vi "hit judge.vi"(6 "keys pressed":T1(array[ring]), 7 "click last frame":T1(array[ring]), 8 "hold note key":T2, 9 "score info":T3, 10 "next note":cluster{"1st rail":i32, "2nd rail":i32}, 11 "song info":T4) -> (0 "hold note key":T2, 1 "new score info":T3, 2 "next note":cluster{"1st rail":i32, "2nd rail":i32}, 3 "note acc":cluster{i32, i32})   [LabVIEW 2023]
panel:
  out "keys pressed 2":T1(array[ring])
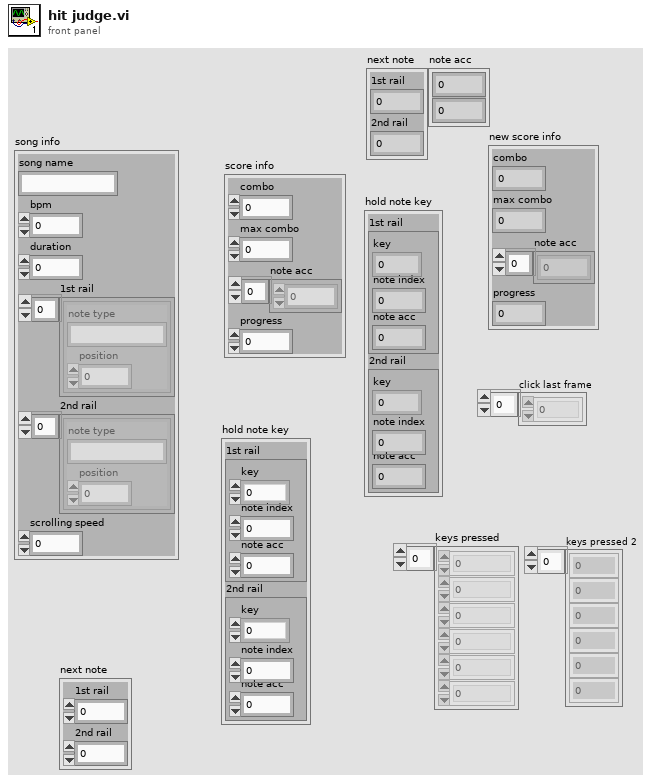
[diagram p1: front panel]
types:
  T1 = enum16{"0", "1", "2", "3", "4", "5", "6", "7", "8", "9", "A", "B", "C", "D", "E", "F", "G", "H", "I", "J", "K", "L", "M", "N", "O", "P", "Q", "R", "S", "T", "U", "V", "W", "X", "Y", "Z", "F1", "F2", "F3", "F4", "F5", "F6", "F7", "F8", "F9", "F10", "F11", "F12", "F13", "F14", "F15", "ADD", "BACK", "BACKSLASH", "CAPITAL", "COMMA", "DECIMAL", "DELETE", "DIVIDE", "DOWN", "END", "EQUALS", "ESCAPE", "GRAVE (`)", "HOME", "INSERT", "LBRACKET", "LCONTROL", "LEFT", "L ALT", "LSHIFT", "LWIN", "MINUS", "MULTIPLY", "NEXT", "NUMLOCK", "NUMPAD_0", "NUMPAD_1", "NUMPAD_2", "NUMPAD_3", "NUMPAD_4", "NUMPAD_5", "NUMPAD_6", "NUMPAD_7", "NUMPAD_8", "NUMPAD_9", "PAUSE", "PERIOD", "PRIOR (PG UP)", "RBRACKET", "RCONTROL", "RETURN", "RIGHT", "R ALT", "RSHIFT", "RWIN", "SCROLL", "SEMICOLON", "SLASH", "SPACE", "SUBTRACT", "TAB", "UP", "ENTER (num pad)", "' (quote)"}[]
  T2 = cluster{"1st rail":cluster{"key":enum16{"0", "1", "2", "3", "4", "5", "6", "7", "8", "9", "A", "B", "C", "D", "E", "F", "G", "H", "I", "J", "K", "L", "M", "N", "O", "P", "Q", "R", "S", "T", "U", "V", "W", "X", "Y", "Z", "F1", "F2", "F3", "F4", "F5", "F6", "F7", "F8", "F9", "F10", "F11", "F12", "F13", "F14", "F15", "ADD", "BACK", "BACKSLASH", "CAPITAL", "COMMA", "DECIMAL", "DELETE", "DIVIDE", "DOWN", "END", "EQUALS", "ESCAPE", "GRAVE (`)", "HOME", "INSERT", "LBRACKET", "LCONTROL", "LEFT", "L ALT", "LSHIFT", "LWIN", "MINUS", "MULTIPLY", "NEXT", "NUMLOCK", "NUMPAD_0", "NUMPAD_1", "NUMPAD_2", "NUMPAD_3", "NUMPAD_4", "NUMPAD_5", "NUMPAD_6", "NUMPAD_7", "NUMPAD_8", "NUMPAD_9", "PAUSE", "PERIOD", "PRIOR (PG UP)", "RBRACKET", "RCONTROL", "RETURN", "RIGHT", "R ALT", "RSHIFT", "RWIN", "SCROLL", "SEMICOLON", "SLASH", "SPACE", "SUBTRACT", "TAB", "UP", "ENTER (num pad)", "' (quote)"}, "note index":i32, "note acc":i32}, "2nd rail":cluster{"key":enum16{"0", "1", "2", "3", "4", "5", "6", "7", "8", "9", "A", "B", "C", "D", "E", "F", "G", "H", "I", "J", "K", "L", "M", "N", "O", "P", "Q", "R", "S", "T", "U", "V", "W", "X", "Y", "Z", "F1", "F2", "F3", "F4", "F5", "F6", "F7", "F8", "F9", "F10", "F11", "F12", "F13", "F14", "F15", "ADD", "BACK", "BACKSLASH", "CAPITAL", "COMMA", "DECIMAL", "DELETE", "DIVIDE", "DOWN", "END", "EQUALS", "ESCAPE", "GRAVE (`)", "HOME", "INSERT", "LBRACKET", "LCONTROL", "LEFT", "L ALT", "LSHIFT", "LWIN", "MINUS", "MULTIPLY", "NEXT", "NUMLOCK", "NUMPAD_0", "NUMPAD_1", "NUMPAD_2", "NUMPAD_3", "NUMPAD_4", "NUMPAD_5", "NUMPAD_6", "NUMPAD_7", "NUMPAD_8", "NUMPAD_9", "PAUSE", "PERIOD", "PRIOR (PG UP)", "RBRACKET", "RCONTROL", "RETURN", "RIGHT", "R ALT", "RSHIFT", "RWIN", "SCROLL", "SEMICOLON", "SLASH", "SPACE", "SUBTRACT", "TAB", "UP", "ENTER (num pad)", "' (quote)"}, "note index":i32, "note acc":i32}}
  T3 = cluster{"combo":i32, "max combo":i32, "note acc":i32[], "progress":dbl}
  T4 = cluster{"song name":string, "bpm":i32, "duration":i32, "1st rail":cluster{"note type":string, "position":dbl}[], "2nd rail":cluster{"note type":string, "position":dbl}[], "scrolling speed":dbl}
  T5 = enum16{"0", "1", "2", "3", "4", "5", "6", "7", "8", "9", "A", "B", "C", "D", "E", "F", "G", "H", "I", "J", "K", "L", "M", "N", "O", "P", "Q", "R", "S", "T", "U", "V", "W", "X", "Y", "Z", "F1", "F2", "F3", "F4", "F5", "F6", "F7", "F8", "F9", "F10", "F11", "F12", "F13", "F14", "F15", "ADD", "BACK", "BACKSLASH", "CAPITAL", "COMMA", "DECIMAL", "DELETE", "DIVIDE", "DOWN", "END", "EQUALS", "ESCAPE", "GRAVE (`)", "HOME", "INSERT", "LBRACKET", "LCONTROL", "LEFT", "L ALT", "LSHIFT", "LWIN", "MINUS", "MULTIPLY", "NEXT", "NUMLOCK", "NUMPAD_0", "NUMPAD_1", "NUMPAD_2", "NUMPAD_3", "NUMPAD_4", "NUMPAD_5", "NUMPAD_6", "NUMPAD_7", "NUMPAD_8", "NUMPAD_9", "PAUSE", "PERIOD", "PRIOR (PG UP)", "RBRACKET", "RCONTROL", "RETURN", "RIGHT", "R ALT", "RSHIFT", "RWIN", "SCROLL", "SEMICOLON", "SLASH", "SPACE", "SUBTRACT", "TAB", "UP", "ENTER (num pad)", "' (quote)"}
  T6 = cluster{"key":enum16{"0", "1", "2", "3", "4", "5", "6", "7", "8", "9", "A", "B", "C", "D", "E", "F", "G", "H", "I", "J", "K", "L", "M", "N", "O", "P", "Q", "R", "S", "T", "U", "V", "W", "X", "Y", "Z", "F1", "F2", "F3", "F4", "F5", "F6", "F7", "F8", "F9", "F10", "F11", "F12", "F13", "F14", "F15", "ADD", "BACK", "BACKSLASH", "CAPITAL", "COMMA", "DECIMAL", "DELETE", "DIVIDE", "DOWN", "END", "EQUALS", "ESCAPE", "GRAVE (`)", "HOME", "INSERT", "LBRACKET", "LCONTROL", "LEFT", "L ALT", "LSHIFT", "LWIN", "MINUS", "MULTIPLY", "NEXT", "NUMLOCK", "NUMPAD_0", "NUMPAD_1", "NUMPAD_2", "NUMPAD_3", "NUMPAD_4", "NUMPAD_5", "NUMPAD_6", "NUMPAD_7", "NUMPAD_8", "NUMPAD_9", "PAUSE", "PERIOD", "PRIOR (PG UP)", "RBRACKET", "RCONTROL", "RETURN", "RIGHT", "R ALT", "RSHIFT", "RWIN", "SCROLL", "SEMICOLON", "SLASH", "SPACE", "SUBTRACT", "TAB", "UP", "ENTER (num pad)", "' (quote)"}, "note index":i32, "note acc":i32}
  T7 = cluster{"element":enum16{"0", "1", "2", "3", "4", "5", "6", "7", "8", "9", "A", "B", "C", "D", "E", "F", "G", "H", "I", "J", "K", "L", "M", "N", "O", "P", "Q", "R", "S", "T", "U", "V", "W", "X", "Y", "Z", "F1", "F2", "F3", "F4", "F5", "F6", "F7", "F8", "F9", "F10", "F11", "F12", "F13", "F14", "F15", "ADD", "BACK", "BACKSLASH", "CAPITAL", "COMMA", "DECIMAL", "DELETE", "DIVIDE", "DOWN", "END", "EQUALS", "ESCAPE", "GRAVE (`)", "HOME", "INSERT", "LBRACKET", "LCONTROL", "LEFT", "L ALT", "LSHIFT", "LWIN", "MINUS", "MULTIPLY", "NEXT", "NUMLOCK", "NUMPAD_0", "NUMPAD_1", "NUMPAD_2", "NUMPAD_3", "NUMPAD_4", "NUMPAD_5", "NUMPAD_6", "NUMPAD_7", "NUMPAD_8", "NUMPAD_9", "PAUSE", "PERIOD", "PRIOR (PG UP)", "RBRACKET", "RCONTROL", "RETURN", "RIGHT", "R ALT", "RSHIFT", "RWIN", "SCROLL", "SEMICOLON", "SLASH", "SPACE", "SUBTRACT", "TAB", "UP", "ENTER (num pad)", "' (quote)"}, i32, i32}
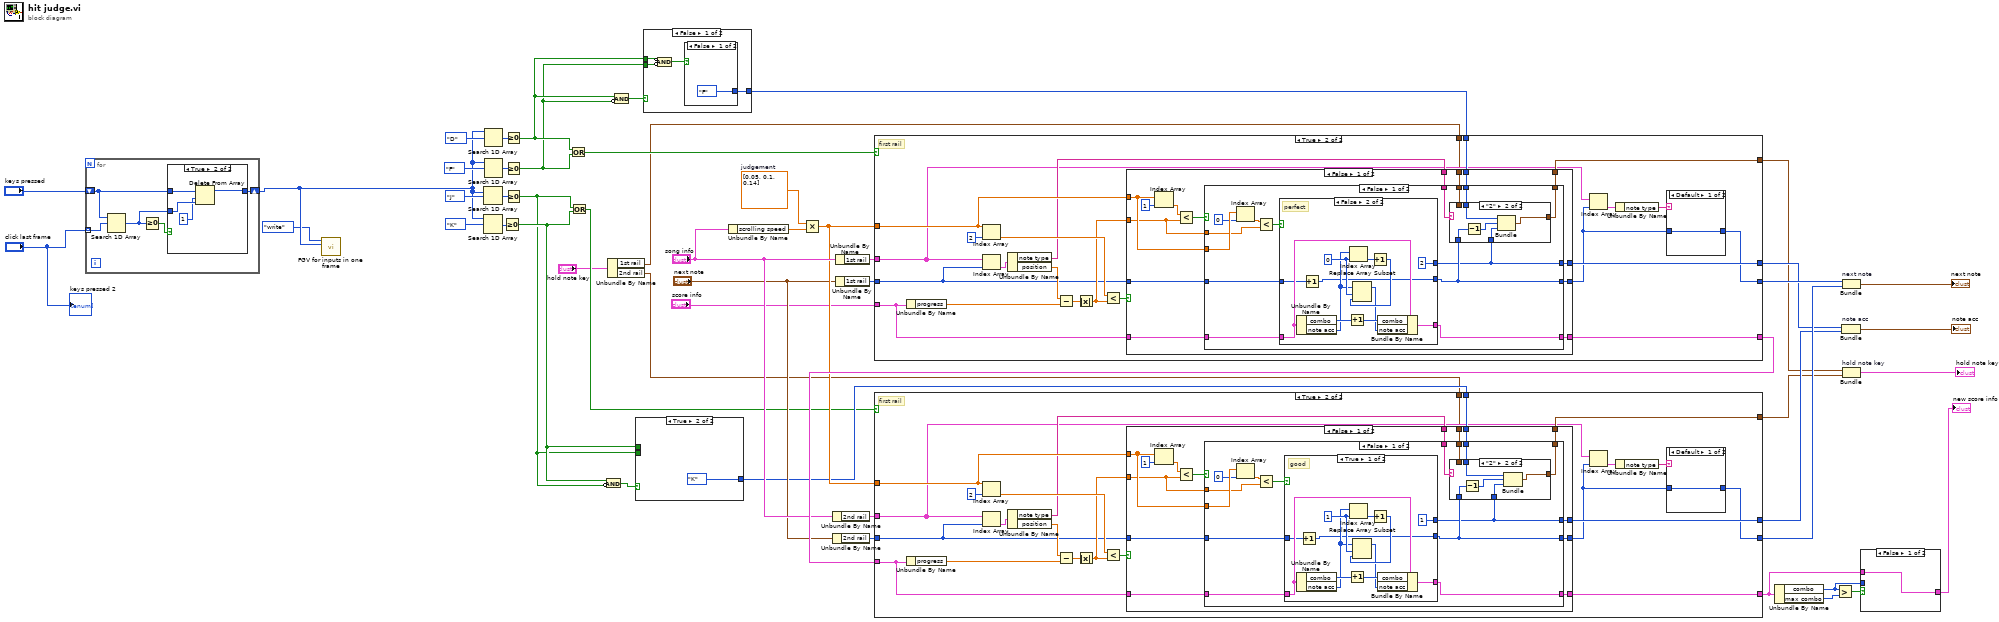
[diagram p0: block diagram]
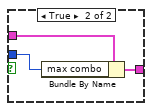
[diagram p3: hidden frame]
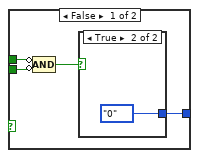
[diagram p4: hidden frame]
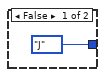
[diagram p5: hidden frame]
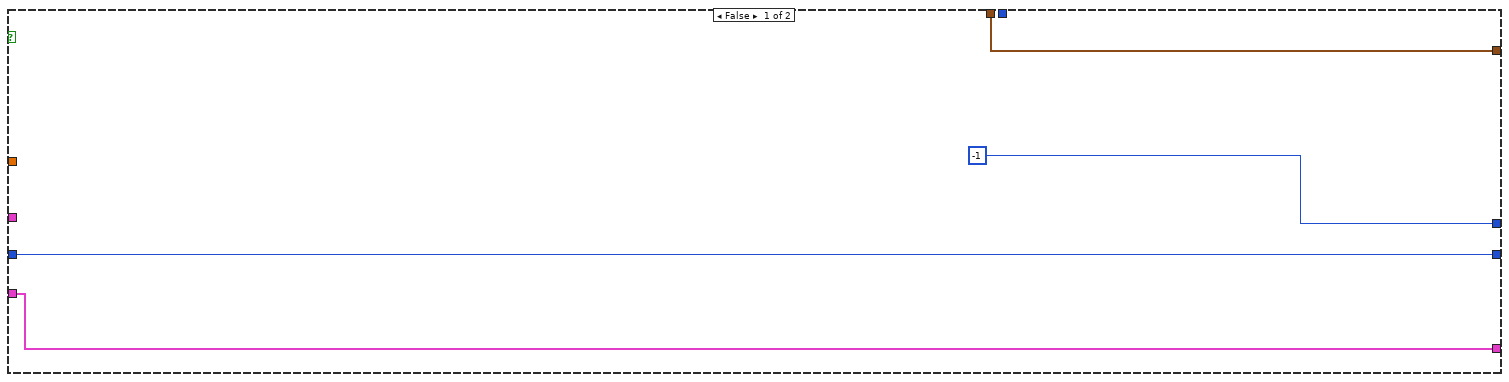
[diagram p6: hidden frame]
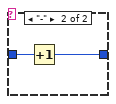
[diagram p7: hidden frame]
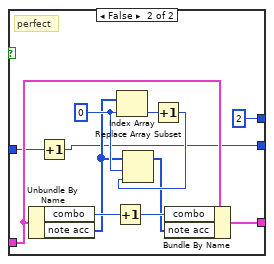
[diagram p9: hidden frame]
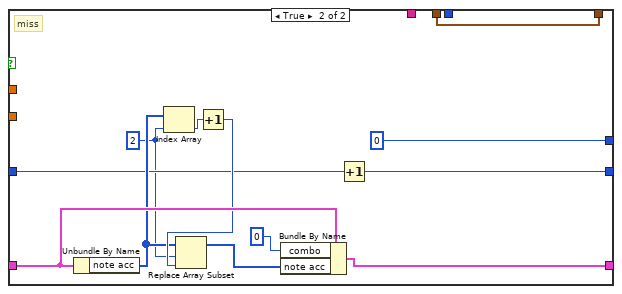
[diagram p10: hidden frame]
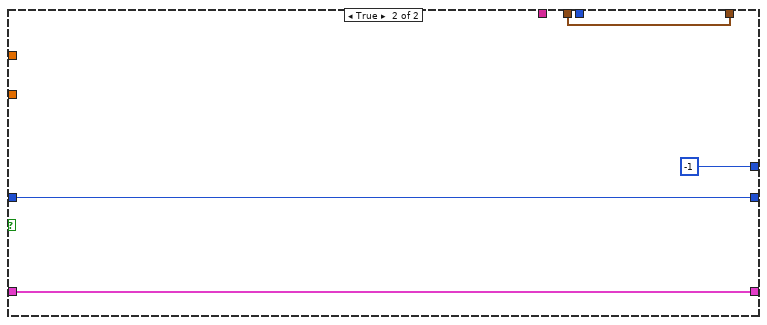
[diagram p11: hidden frame]
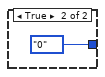
[diagram p12: hidden frame]
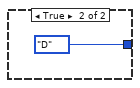
[diagram p13: hidden frame]
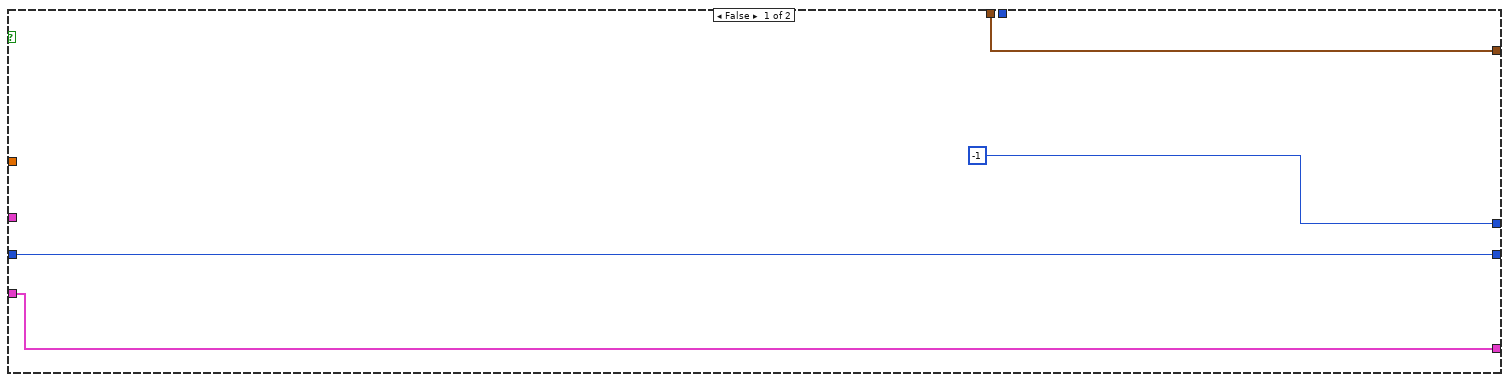
[diagram p14: hidden frame]
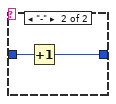
[diagram p15: hidden frame]
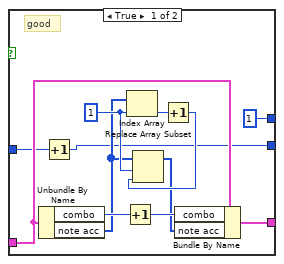
[diagram p17: hidden frame]
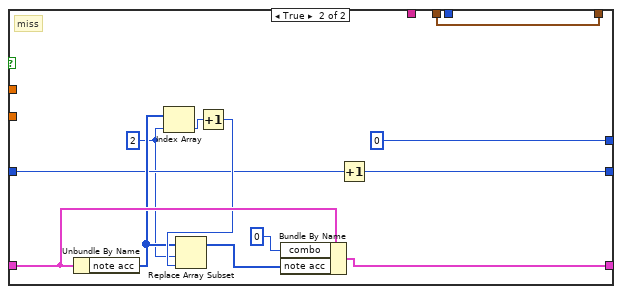
[diagram p18: hidden frame]
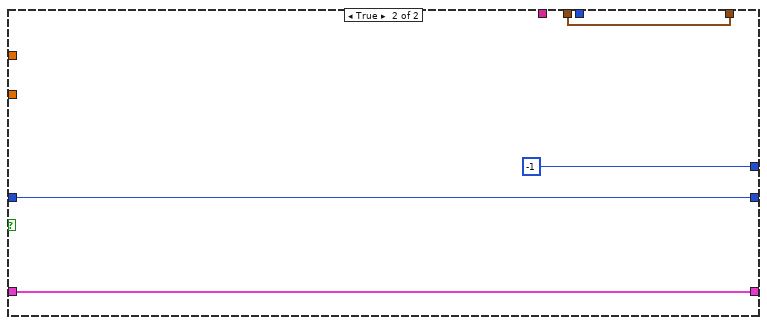
[diagram p19: hidden frame]
diagram:
  w49 = dbl[] [0.05, 0.1, 0.14]  # judgement
  n1 = for {
    tunnel: "click last frame" -> [w55] mode=indexing
    shift-right: [w52] -> w3
    shift-left: "keys pressed" -> [w53]
    n2 = Search 1D Array(1D array=w53, element=w55) -> (index of element=w51:i32)  [unwired: 1 in]
    n3 = Greater Or Equal To 0?(x=w51) -> (x >= 0?=w54:bool)
    n4 = case shown="True" w54 {
      tunnel: w53 -> [w56 w60]
      tunnel: [w56 w59] -> w52
      tunnel: w51 -> [_ w58]
      frame False {
      }
      frame True {
        n5 = Delete From Array(array=w60, length=1, index=w58) -> (array with subset deleted=w59:T1)  [unwired: 1 out]
      }
    }
  }
  n6 = call "FGV for inputs in one frame.vi"("write in key"=w3, "mode"=enum16{"read", "write"}."write") -> ()  [unwired: 9 in, 1 out]
  n7 = Search 1D Array(1D array=w3, element=T5."J") -> (index of element=w42:i32)  [unwired: 1 in]
  n8 = Search 1D Array(1D array=w3, element=T5."K") -> (index of element=w41:i32)  [unwired: 1 in]
  n9 = Search 1D Array(1D array=w3, element=T5."D") -> (index of element=w46:i32)  [unwired: 1 in]
  n10 = Search 1D Array(1D array=w3, element=T5."F") -> (index of element=w45:i32)  [unwired: 1 in]
  n11 = Greater Or Equal To 0?(x=w41) -> (x >= 0?=w26:bool)
  n12 = Greater Or Equal To 0?(x=w46) -> (x >= 0?=w37:bool)
  n13 = Greater Or Equal To 0?(x=w45) -> (x >= 0?=w36:bool)
  n14 = Greater Or Equal To 0?(x=w42) -> (x >= 0?=w25:bool)
  n15 = Or(x=w37, y=w36) -> (x .or. y?=w40:bool)
  n16 = Or(x=w25, y=w26) -> (x .or. y?=w23:bool)
  n17 = Compound Arithmetic op=AND(w26, invert w25) -> (w27:bool)
  n18 = Unbundle By Name("hold note key") -> ("1st rail"=w6:T6, "2nd rail"=w5:T6)
  n19 = Compound Arithmetic op=AND(w37, invert w36) -> (w38:bool)
  n20 = case shown="True" w27 {
    tunnel: [w61 T5."K" ("element")] -> w24
    tunnel: w26 -> [w64 _]
    tunnel: w25 -> [w63 _]
    frame False {
      n21 = Compound Arithmetic op=AND(invert w64, invert w63) -> (w62:bool)
      n22 = case shown="True" w62 {
        tunnel: [T5."J" ("element") T5."0" ("element")] -> w61
        frame False {
        }
        frame True {
        }
      }
    }
    frame True {
    }
  }
  n23 = case shown="False" w38 {
    tunnel: [w68 T5."D" ("element")] -> w35
    tunnel: w37 -> [w71 _]
    tunnel: w36 -> [w70 _]
    frame False {
      n24 = Compound Arithmetic op=AND(invert w71, invert w70) -> (w69:bool)
      n25 = case shown="False" w69 {
        tunnel: [T5."F" ("element") T5."0" ("element")] -> w68
        frame False {
        }
        frame True {
        }
      }
    }
    frame True {
    }
  }
  n26 = Unbundle By Name("song info") -> ("scrolling speed"=w50:dbl)
  n27 = Multiply(x=w49, y=w50) -> (x*y=w32:dbl[])
  n28 = Unbundle By Name("song info") -> ("2nd rail"=w28:cluster{"note type":string, "position":dbl}[])
  n29 = Unbundle By Name("next note") -> ("2nd rail"=w30:i32)
  n30 = Unbundle By Name("song info") -> ("1st rail"=w29:cluster{"note type":string, "position":dbl}[])
  n31 = Unbundle By Name("next note") -> ("1st rail"=w39:i32)
  n32 = case shown="True" w40 {
    tunnel: w32 -> [_ w91]
    tunnel: "score info" -> [w78 w93]
    tunnel: [w78 w92] -> w34
    tunnel: [w77 w81] -> w22
    tunnel: w39 -> [w77 w89]
    tunnel: [-1 w88] -> w20
    tunnel: w35 -> [_ w86]
    tunnel: w6 -> [w75 w79]
    tunnel: [w75 w85] -> w18
    tunnel: w29 -> [_ w80]
    frame False {
    }
    frame True {
      # "first rail"
      n33 = Unbundle By Name(w93) -> ("progress"=w97:dbl)
      n34 = Index Array(array=w91, index=2) -> (element=w94:dbl)
      n35 = Index Array(array=w80, index=w89) -> (element=w100:cluster{"note type":string, "position":dbl})
      n36 = Unbundle By Name(w100) -> ("note type"=w87:string, "position"=w98:dbl)
      n37 = Subtract(x=w98, y=w97) -> (x-y=w96:dbl)
      n38 = Absolute Value(x=w96) -> (abs(x)=w90:dbl)
      n39 = Less?(x=w94, y=w90) -> (x < y?=w95:bool)
      n40 = case shown="False" w95 {
        tunnel: w89 -> [w111 w177]
        tunnel: w93 -> [w114 w176]
        tunnel: [w113 w176] -> w92
        tunnel: [w112 w177] -> w82
        tunnel: w91 -> [w110 _]
        tunnel: w90 -> [w109 _]
        tunnel: [w108 -1] -> w88
        tunnel: w87 -> [w107 _]
        tunnel: w86 -> [w106 _]
        tunnel: [w105 w174] -> w85
        tunnel: w79 -> [w104 w174]
        frame False {
          n41 = Index Array(array=w110, index=1) -> (element=w116:dbl)
          n42 = Less?(x=w116, y=w109) -> (x < y?=w115:bool)
          n43 = case shown="False" w115 {
            tunnel: w114 -> [w126 w173]
            tunnel: [w125 w172] -> w113
            tunnel: [w120 w166] -> w112
            tunnel: w111 -> [w124 w165]
            tunnel: w110 -> [w131 _]
            tunnel: w109 -> [w129 _]
            tunnel: [w118 0] -> w108
            tunnel: w107 -> [w123 _]
            tunnel: w106 -> [w122 _]
            tunnel: [w121 w162] -> w105
            tunnel: w104 -> [w119 w162]
            frame False {
              n44 = Index Array(array=w131, index=0) -> (element=w128:dbl)
              n45 = Less?(x=w128, y=w129) -> (x < y?=w127:bool)
              n46 = case shown="False" w127 {
                tunnel: w126 -> [w149 w161]
                tunnel: [w148 w160] -> w125
                tunnel: w124 -> [w140 w152]
                tunnel: [w139 w151] -> w120
                tunnel: [1 2] -> w118
                frame True {
                  w144 = 1
                  # "good"
                  n47 = Unbundle By Name(w149) -> ("combo"=w146:i32, "note acc"=w143:i32[])
                  n48 = Increment(x=w140) -> (x+1=w139:i32)
                  n49 = Increment(x=w146) -> (x+1=w147:i32)
                  n50 = Index Array(array=w143, index=w144) -> (element=w145:i32)
                  n51 = Increment(x=w145) -> (x+1=w142:i32)
                  n52 = Replace Array Subset(array=w143, new element=w142, index=w144) -> (w141:i32[])
                  n53 = Bundle By Name(cluster=w149, "combo"=w147, "note acc"=w141) -> (w148:T3)
                }
                frame False {
                  w156 = 0
                  # "perfect"
                  n54 = Unbundle By Name(w161) -> ("combo"=w158:i32, "note acc"=w155:i32[])
                  n55 = Increment(x=w152) -> (x+1=w151:i32)
                  n56 = Increment(x=w158) -> (x+1=w159:i32)
                  n57 = Index Array(array=w155, index=w156) -> (element=w157:i32)
                  n58 = Increment(x=w157) -> (x+1=w154:i32)
                  n59 = Replace Array Subset(array=w155, new element=w154, index=w156) -> (w153:i32[])
                  n60 = Bundle By Name(cluster=w161, "combo"=w159, "note acc"=w153) -> (w160:T3)
                }
              }
              n61 = case shown="\"2\"" w123 {
                tunnel: [w132 w136] -> w121
                tunnel: w122 -> [_ w134]
                tunnel: w120 -> [_ w137]
                tunnel: w119 -> [w132 _]
                tunnel: w118 -> [_ w133]
                frame Default {
                }
                frame "2" {
                  n62 = Decrement(x=w137) -> (x-1=w135:i32)
                  n63 = Bundle("element"=w134, w135, w133) -> (w136:T7)  [unwired: 1 in]
                }
              }
            }
            frame True {
              w164 = 2 ("new element/subarray")
              # "miss"
              n64 = Unbundle By Name(w173) -> ("note acc"=w168:i32[])
              n65 = Index Array(array=w168, index=w164) -> (element=w170:i32)
              n66 = Increment(x=w170) -> (x+1=w169:i32)
              n67 = Replace Array Subset(array=w168, new element=w169, index=w164) -> (w167:i32[])
              n68 = Bundle By Name(cluster=w173, "combo"=0, "note acc"=w167) -> (w172:T3)
              n69 = Increment(x=w165) -> (x+1=w166:i32)
            }
          }
        }
        frame True {
        }
      }
      n70 = Index Array(array=w80, index=w82) -> (element=w84:cluster{"note type":string, "position":dbl})
      n71 = Unbundle By Name(w84) -> ("note type"=w83:string)
      n72 = case shown="Default" w83 {
        tunnel: w82 -> [w101 w103]
        tunnel: [w101 w102] -> w81
        frame Default {
        }
        frame "-" {
          n73 = Increment(x=w103) -> (x+1=w102:i32)
        }
      }
    }
  }
  n74 = case shown="True" w23 {
    tunnel: w32 -> [_ w194]
    tunnel: w34 -> [w181 w196]
    tunnel: [w181 w195] -> w11
    tunnel: [w180 w184] -> w21
    tunnel: w30 -> [w180 w192]
    tunnel: [-1 w191] -> w19
    tunnel: w24 -> [_ w189]
    tunnel: w5 -> [w178 w182]
    tunnel: [w178 w188] -> w17
    tunnel: w28 -> [_ w183]
    frame False {
    }
    frame True {
      # "first rail"
      n75 = Unbundle By Name(w196) -> ("progress"=w200:dbl)
      n76 = Index Array(array=w194, index=2) -> (element=w197:dbl)
      n77 = Index Array(array=w183, index=w192) -> (element=w203:cluster{"note type":string, "position":dbl})
      n78 = Unbundle By Name(w203) -> ("note type"=w190:string, "position"=w201:dbl)
      n79 = Subtract(x=w201, y=w200) -> (x-y=w199:dbl)
      n80 = Absolute Value(x=w199) -> (abs(x)=w193:dbl)
      n81 = Less?(x=w197, y=w193) -> (x < y?=w198:bool)
      n82 = case shown="False" w198 {
        tunnel: w192 -> [w214 w280]
        tunnel: w196 -> [w217 w279]
        tunnel: [w216 w279] -> w195
        tunnel: [w215 w280] -> w185
        tunnel: w194 -> [w213 _]
        tunnel: w193 -> [w212 _]
        tunnel: [w211 -1] -> w191
        tunnel: w190 -> [w210 _]
        tunnel: w189 -> [w209 _]
        tunnel: [w208 w277] -> w188
        tunnel: w182 -> [w207 w277]
        frame False {
          n83 = Index Array(array=w213, index=1) -> (element=w219:dbl)
          n84 = Less?(x=w219, y=w212) -> (x < y?=w218:bool)
          n85 = case shown="False" w218 {
            tunnel: w217 -> [w229 w276]
            tunnel: [w228 w275] -> w216
            tunnel: [w223 w269] -> w215
            tunnel: w214 -> [w227 w268]
            tunnel: w213 -> [w234 _]
            tunnel: w212 -> [w232 _]
            tunnel: [w221 0] -> w211
            tunnel: w210 -> [w226 _]
            tunnel: w209 -> [w225 _]
            tunnel: [w224 w265] -> w208
            tunnel: w207 -> [w222 w265]
            frame False {
              n86 = Index Array(array=w234, index=0) -> (element=w231:dbl)
              n87 = Less?(x=w231, y=w232) -> (x < y?=w230:bool)
              n88 = case shown="True" w230 {
                tunnel: w229 -> [w252 w264]
                tunnel: [w251 w263] -> w228
                tunnel: w227 -> [w243 w255]
                tunnel: [w242 w254] -> w223
                tunnel: [1 2] -> w221
                frame True {
                  w247 = 1
                  # "good"
                  n89 = Unbundle By Name(w252) -> ("combo"=w249:i32, "note acc"=w246:i32[])
                  n90 = Increment(x=w243) -> (x+1=w242:i32)
                  n91 = Increment(x=w249) -> (x+1=w250:i32)
                  n92 = Index Array(array=w246, index=w247) -> (element=w248:i32)
                  n93 = Increment(x=w248) -> (x+1=w245:i32)
                  n94 = Replace Array Subset(array=w246, new element=w245, index=w247) -> (w244:i32[])
                  n95 = Bundle By Name(cluster=w252, "combo"=w250, "note acc"=w244) -> (w251:T3)
                }
                frame False {
                  w259 = 0
                  # "perfect"
                  n96 = Unbundle By Name(w264) -> ("combo"=w261:i32, "note acc"=w258:i32[])
                  n97 = Increment(x=w255) -> (x+1=w254:i32)
                  n98 = Increment(x=w261) -> (x+1=w262:i32)
                  n99 = Index Array(array=w258, index=w259) -> (element=w260:i32)
                  n100 = Increment(x=w260) -> (x+1=w257:i32)
                  n101 = Replace Array Subset(array=w258, new element=w257, index=w259) -> (w256:i32[])
                  n102 = Bundle By Name(cluster=w264, "combo"=w262, "note acc"=w256) -> (w263:T3)
                }
              }
              n103 = case shown="\"2\"" w226 {
                tunnel: [w235 w237] -> w224
                tunnel: w225 -> [_ w239]
                tunnel: w223 -> [_ w240]
                tunnel: w222 -> [w235 _]
                tunnel: w221 -> [_ w236]
                frame Default {
                }
                frame "2" {
                  n104 = Decrement(x=w240) -> (x-1=w238:i32)
                  n105 = Bundle("element"=w239, w238, w236) -> (w237:T7)  [unwired: 1 in]
                }
              }
            }
            frame True {
              w267 = 2 ("new element/subarray")
              # "miss"
              n106 = Unbundle By Name(w276) -> ("note acc"=w271:i32[])
              n107 = Index Array(array=w271, index=w267) -> (element=w273:i32)
              n108 = Increment(x=w273) -> (x+1=w272:i32)
              n109 = Replace Array Subset(array=w271, new element=w272, index=w267) -> (w270:i32[])
              n110 = Bundle By Name(cluster=w276, "combo"=0, "note acc"=w270) -> (w275:T3)
              n111 = Increment(x=w268) -> (x+1=w269:i32)
            }
          }
        }
        frame True {
        }
      }
      n112 = Index Array(array=w183, index=w185) -> (element=w187:cluster{"note type":string, "position":dbl})
      n113 = Unbundle By Name(w187) -> ("note type"=w186:string)
      n114 = case shown="Default" w186 {
        tunnel: w185 -> [w204 w206]
        tunnel: [w204 w205] -> w184
        frame Default {
        }
        frame "-" {
          n115 = Increment(x=w206) -> (x+1=w205:i32)
        }
      }
    }
  }
  n116 = Unbundle By Name(w11) -> ("combo"=w10:i32, "max combo"=w13:i32)
  n117 = Greater?(x=w10, y=w13) -> (0:w12:bool)
  n118 = Bundle "note acc"(w20, w19) -> (→"note acc":cluster{i32, i32})  [unwired: 1 in]
  n119 = Bundle "next note"("1st rail"=w22, "2nd rail"=w21) -> (→"next note":cluster{"1st rail":i32, "2nd rail":i32})  [unwired: 1 in]
  n120 = Bundle "hold note key"("1st rail"=w18, "2nd rail"=w17) -> (→"hold note key":T2)  [unwired: 1 in]
  n121 = case shown="False" w12 {
    tunnel: w11 -> [w281 w284]
    tunnel: w10 -> [_ w283]
    tunnel: [w281 w282] -> w9
    frame False {
    }
    frame True {
      n122 = Bundle By Name(cluster=w284, "max combo"=w283) -> (w282:T3)
    }
  }
  "new score info" <- w9
  "keys pressed 2" <- "click last frame"
